vi "Parse Group Parameters and Log.vi"(8 "error in":errorcluster, 10 "Variant":variant, 11 "Report in":refnum<class "Report.lvclass">) -> (0 "error out":errorcluster, 3 "Report out":refnum<class "Report.lvclass">)   [LabVIEW 2023, in "Report.lvlib" / "Report.lvclass"]
doc: "This VI takes a variant containing a group name, an array of string parameter descriptors and an array of variant parameter values. \n\nThe parameters are logged to the group properties to be read back in post processing."
uses:
  Report.lvclass
  Custom Controls/Report Action.ctl
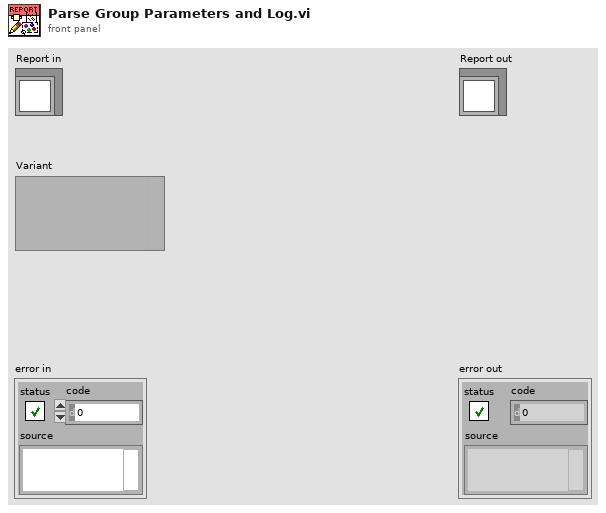
[diagram p1: front panel]
types:
  T1 = typedef "Report.lvlib/Report.lvclass/Report Action.ctl" = enum16{"Create", "Append", "Destroy"}
  T2 = cluster{"Group":string, "Properties":string[], "Values":variant[]}
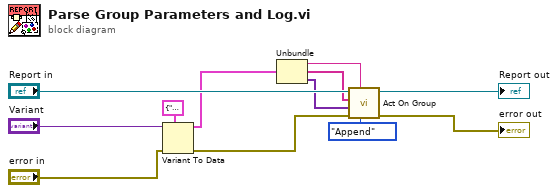
[diagram p0: block diagram]
diagram:
  n1 = Variant To Data(error in="error in", type=T2 {"Group"="", "Properties"=[], "Values"=[]} ("NChanMsg"), Variant="Variant") -> (data=w7:T2, error out=w8:errorcluster)
  n2 = Unbundle(w7) -> ("Group"=w6:string, "Properties"=w5:string[], "Values"=w4:variant[])
  n3 = call-dynamic "Act On Group.vi"("Report Action"=Report_Action."Append", "Group Name"=w6, "error in (no error)"=w8, "Values"=w4, "Parameters"=w5, "Report in"="Report in") -> ("error out"=→"error out":errorcluster, "Report out"=→"Report out":refnum<class "Report.lvclass">)  [unwired: 4 in]
